vi "Read Latest Value as Variant.vi"(8 "error in (no error)":errorcluster, 10 "index":i32[](array[numeric]), 11 "Ring Buffer":T1) -> (0 "error out":errorcluster, 1 "Values":variant, 2 "Timestamps":u64, 3 "Ring Buffer":T1)   [LabVIEW 2021, in "Ring Buffer Strict Accessor.lvlib"]
uses:
  Ring Buffer Strict Accessor.lvlib
  SubVIs/RingBufferHandle.ctl
  <userlib>/bjustice/Ring Buffer for Time Series Data/SubVIs/DVR data.ctl
  SubVIs/DataType.ctl
  SubVIs/Endianess.ctl
  <userlib>/bjustice/Ring Buffer for Time Series Data/API/Read Latest Value.vi
  <userlib>/bjustice/Ring Buffer for Time Series Data/SubVIs/Newest Value Index.vi
  <userlib>/bjustice/Ring Buffer for Time Series Data/SubVIs/empty buffer check.vi
  SubVIs/datatype byte size.vi
  SubVIs/array sizes to number of points.vi
  SubVIs/ByteArray to Variant.vi/8a60398d-b755-4916-b991-d3a0bc5f0417.vi
  SubVIs/ByteArray to Variant.vi/751c3a01-ff04-4836-b7a6-7b574d4a9b81.vi
  SubVIs/ByteArray to Variant.vi/221f450a-1b6f-46a4-a2fc-afe85f1524e2.vi
  SubVIs/ByteArray to Variant.vi/41001614-cdbd-4ebb-921a-864de9ec47e2.vi
  SubVIs/ByteArray to Variant.vi/5546051e-c623-4301-8272-f4bdabd7954b.vi
  SubVIs/ByteArray to Variant.vi/5ca96b41-1aac-43f3-81c4-abd3cf1c6587.vi
  SubVIs/ByteArray to Variant.vi/7d34a3b6-a7c4-49dd-9cdf-fb0f78c178d5.vi
  SubVIs/ByteArray to Variant.vi/d8189c62-4619-451b-9af1-1c592367667c.vi
  SubVIs/ByteArray to Variant.vi/ae543023-a94a-4a2d-bef6-e89c8b6f7eb3.vi
  SubVIs/ByteArray to Variant.vi/788b2cc3-569e-4ae0-be57-2fef15c96938.vi
  SubVIs/ByteArray to Variant.vi/2b477ad7-803c-4946-b2f4-1fc748402100.vi
  SubVIs/ByteArray to Variant.vi/098c5dbb-e4d0-4c7a-81ed-dc9b4f9ca07a.vi
  SubVIs/ByteArray to Variant.vi/0e7c8b9e-e897-4ed3-8864-39927aea5c8f.vi
  SubVIs/ByteArray to Variant.vi/f4fc8823-9e07-4dc6-8a2a-c00e5aad4daa.vi
  SubVIs/ByteArray to Variant.vi/4e00dd29-4a4f-4c51-b5d6-93aa465532c5.vi
  SubVIs/ByteArray to Variant.vi/5f2f642a-ad03-4c41-b5d5-f276612f3591.vi
  SubVIs/ByteArray to Variant.vi/571e8695-7815-4b46-9fe8-94e034d2cc8e.vi
  SubVIs/ByteArray to Variant.vi/3d662265-0079-46bb-92db-c9b066d77669.vi
  SubVIs/ByteArray to Variant.vi/817a4f5e-2c65-4066-9894-ecba4a0e477b.vi
  SubVIs/ByteArray to Variant.vi/3fadb452-1f1f-455e-89f0-d18ad6ef6ba2.vi
  SubVIs/ByteArray to Variant.vi/5d6b12d9-691a-45b4-9c34-a3da6780b00a.vi
  SubVIs/ByteArray to Variant.vi/9891769e-6c37-4b59-a094-aa89e879cb8b.vi
  <vilib>/Utility/error.llb/Error Cluster From Error Code.vi
  <userlib>/bjustice/Ring Buffer for Time Series Data/Ring Buffer Time Series Data.lvlib
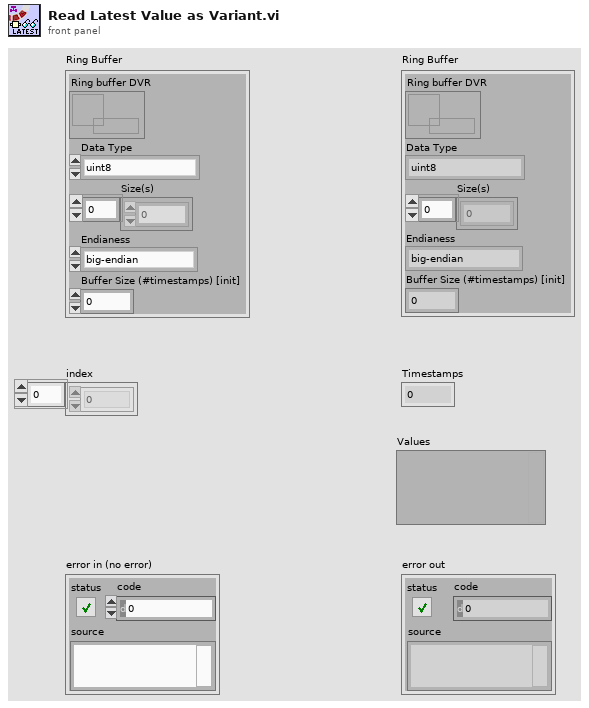
[diagram p1: front panel]
types:
  T1 = typedef "Ring Buffer Strict Accessor.lvlib/RingBufferHandle.ctl" = cluster{"Ring buffer DVR":refnum<data-value>, "Data Type":T2, "Size(s)":i32[], "Endianess":T3, "Buffer Size (#timestamps) [init]":i32}
  T2 = typedef "Ring Buffer Strict Accessor.lvlib/DataType.ctl" = enum16{"uint8", "uint16", "uint32", "uint64", "int8", "int16", "int32", "int64", "float", "double", "extended"}
  T3 = typedef "Ring Buffer Strict Accessor.lvlib/Endianess.ctl" = enum16{"big-endian", "little-endian"}
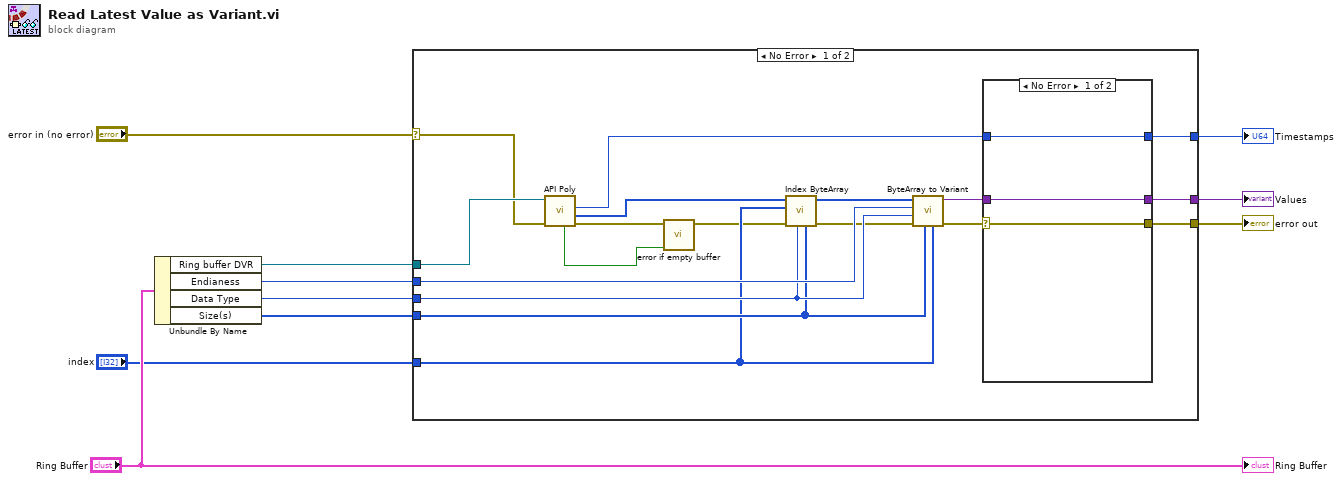
[diagram p0: block diagram]
diagram:
  n1 = Unbundle By Name("Ring Buffer") -> ("Ring buffer DVR"=w8:refnum<data-value>, "Endianess"=w10:T3, "Data Type"=w6:T2, "Size(s)"=w4:i32[])
  n2 = case shown="No Error" "error in (no error)" {
    selector: "error in (no error)" -> [w27 w33]
    tunnel: w10 -> [w21 _]
    tunnel: [w25 _] -> w9
    tunnel: w8 -> [w28 _]
    tunnel: [w26 _] -> w7
    tunnel: w6 -> [w20 _]
    tunnel: [w11 w33] -> w5
    tunnel: w4 -> [w18 _]
    tunnel: "index" -> [w16 _]
    frame No Error {
      n3 = call-poly <userlib>:"API Poly.vi"("error in (no error)"=w27, "Ring buffer DVR in"=w28) -> ("error out"=w15:errorcluster, "Values"=w23:u8[], "Timestamp"=w24:u64, "empty buffer?"=w13:bool)  [unwired: 5 in, 1 out]
      n4 = call "error if empty buffer.vi"("empty buffer?"=w13, "error in (no error)"=w15) -> ("error out"=w14:errorcluster)  [unwired: 9 in]
      n5 = call "Index ByteArray.vi"("Size(s)"=w18, "Data Type"=w20, "error in (no error)"=w14, "index"=w16, "values"=w23) -> ("error out"=w19:errorcluster, "values (indexed)"=w22:u8[])  [unwired: 5 in]
      n6 = call "ByteArray to Variant.vi"("index"=w16, "Size(s)"=w18, "error in (no error)"=w19, "Data Type"=w20, "Endianess"=w21, "byte array"=w22) -> ("error out"=w12:errorcluster, "Variant"=w17:variant)  [unwired: 4 in]
      n7 = case shown="No Error" w12 {
        selector: w12 -> [w29 w32]
        tunnel: w24 -> [w31 _]
        tunnel: [w31 _] -> w26
        tunnel: w17 -> [w30 _]
        tunnel: [w30 _] -> w25
        tunnel: [w29 w32] -> w11
        frame No Error {
        }
        frame Error {
        }
      }
    }
    frame Error {
    }
  }
  "Values" <- w9
  "Timestamps" <- w7
  "error out" <- w5
  "Ring Buffer" <- "Ring Buffer"
